vi "Read UTC Time For String Format.vi"(8 "error in (no error)":errorcluster, 11 "Time in":refnum<class "Abs_Time.lvclass">) -> (0 "error out":errorcluster, 2 "UTC Time For String Format":bool, 3 "Time out":refnum<class "Abs_Time.lvclass">)   [LabVIEW 2021, in "Abs_Time.lvclass"]
uses:
  Abs_Time.lvclass
  Abs_Time.lvclass/Abs_Time.ctl
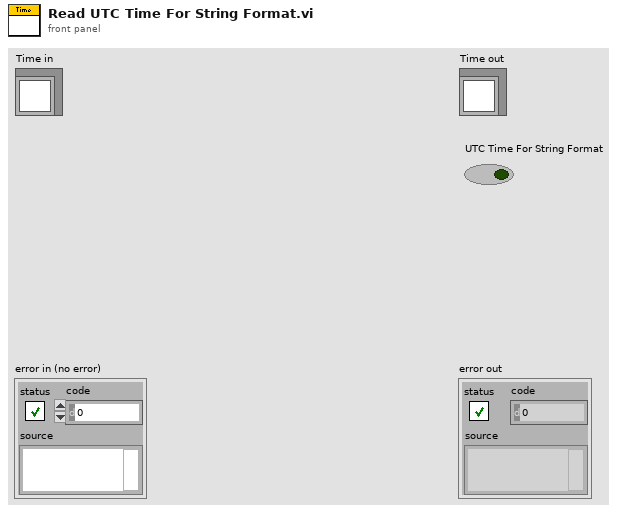
[diagram p1: front panel]
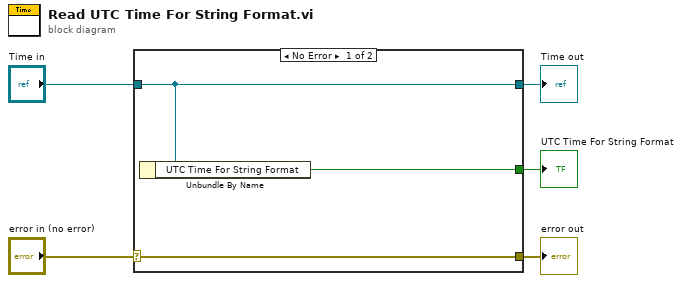
[diagram p0: block diagram]
diagram:
  n1 = case shown="No Error" "error in (no error)" {
    selector: "error in (no error)" -> [w8 w9]
    tunnel: [w8 w9] -> w4
    tunnel: [w7 w10] -> w2
    tunnel: "Time in" -> [w7 w10]
    tunnel: [w6 _] -> w1
    frame No Error {
      n2 = Unbundle By Name(w7) -> ("UTC Time For String Format"=w6:bool)
    }
    frame Error {
    }
  }
  "error out" <- w4
  "Time out" <- w2
  "UTC Time For String Format" <- w1
